vi "holonomic-drive-test.vi"() -> (3 "ALL TESTS PASSED":bool)   [LabVIEW 2019]
uses:
  <vilib>/Rock Robotics/WPI/ThirdParty/JAS_Junk/TrajLib/POSE2D.ctl
  <vilib>/Rock Robotics/WPI/ThirdParty/JAS_Junk/TrajLib/TRANSLATION2D.ctl
  <vilib>/Rock Robotics/WPI/ThirdParty/JAS_Junk/TrajLib/ROTATION2D.ctl
  <vilib>/Rock Robotics/WPI/ThirdParty/JAS_Junk/TrajLib/Translation_Create.vi
  <vilib>/Rock Robotics/WPI/ThirdParty/JAS_Junk/TrajLib/ProfiledPIDController_NewPeriod.vi
  <vilib>/Rock Robotics/WPI/ThirdParty/JAS_Junk/TrajLib/PIDController_NewPeriod.vi
  <vilib>/Rock Robotics/WPI/ThirdParty/JAS_Junk/TrajLib/ProfiledPIDController_Calculate_Meas_Goal.vi
  <vilib>/Rock Robotics/WPI/ThirdParty/JAS_Junk/TrajLib/ChassisSpeeds_FromFieldRelativeSpeeds.vi
  <vilib>/Rock Robotics/WPI/ThirdParty/JAS_Junk/TrajLib/PIDController_Reset.vi
  <vilib>/Rock Robotics/WPI/ThirdParty/JAS_Junk/TrajLib/PIDController_Calculate_SP_PV.vi
  <vilib>/Rock Robotics/WPI/ThirdParty/JAS_Junk/TrajLib/ProfiledPIDController_Reset_PosOnly.vi
  <vilib>/Rock Robotics/WPI/ThirdParty/JAS_Junk/TrajLib/Rotation_GetAngleCosSin.vi
  <vilib>/Rock Robotics/WPI/ThirdParty/JAS_Junk/TrajLib/Pose_RelativeTo.vi
  <vilib>/Rock Robotics/WPI/ThirdParty/JAS_Junk/TrajLib/Pose_getRotation.vi
  <vilib>/Rock Robotics/WPI/ThirdParty/JAS_Junk/TrajLib/Rotation_Minus.vi
  <vilib>/Rock Robotics/WPI/ThirdParty/JAS_Junk/TrajLib/TrapProfState_New.vi
  <vilib>/Rock Robotics/SystemInterfaces/NetworkCommunication/NetComm_UsageReport_report.vi
  <vilib>/Rock Robotics/WPI/ThirdParty/JAS_Junk/TrajLib/ProfiledPIDController_SetGoal_PosOnly.vi
  <vilib>/Rock Robotics/WPI/ThirdParty/JAS_Junk/TrajLib/ProfiledPIDController_Calculate_Meas.vi
  <vilib>/Rock Robotics/WPI/ThirdParty/JAS_Junk/TrajLib/Rotation_GetCos.vi
  <vilib>/Rock Robotics/WPI/ThirdParty/JAS_Junk/TrajLib/Rotation_GetSin.vi
  <vilib>/Rock Robotics/WPI/ThirdParty/JAS_Junk/TrajLib/ChassisSpeeds_New.vi
  <vilib>/Rock Robotics/WPI/ThirdParty/JAS_Junk/TrajLib/PIDController_SetSetpoint.vi
  <vilib>/Rock Robotics/WPI/ThirdParty/JAS_Junk/TrajLib/PIDController_Calculate_PV.vi
  <vilib>/Rock Robotics/WPI/ThirdParty/JAS_Junk/TrajLib/ProfiledPIDController_Reset.vi
  <vilib>/Rock Robotics/WPI/ThirdParty/JAS_Junk/TrajLib/Transform_Create_PosePose.vi
  <vilib>/Rock Robotics/WPI/ThirdParty/JAS_Junk/TrajLib/Pose_New_TRRO.vi
  <vilib>/Rock Robotics/WPI/ThirdParty/JAS_Junk/TrajLib/Rotation_UnaryMinus.vi
  <vilib>/Rock Robotics/WPI/ThirdParty/JAS_Junk/TrajLib/Rotation_RotateBy.vi
  <vilib>/Rock Robotics/WPI/ThirdParty/JAS_Junk/TrajLib/ProfiledPIDController_SetGoal.vi
  <vilib>/Rock Robotics/WPI/ThirdParty/JAS_Junk/TrajLib/TrapProfile_New.vi
  <vilib>/Rock Robotics/WPI/ThirdParty/JAS_Junk/TrajLib/ProfiledPIDController_GetPeriod.vi
  <vilib>/Rock Robotics/WPI/ThirdParty/JAS_Junk/TrajLib/TrapProfile_Calculate.vi
  <vilib>/Rock Robotics/WPI/ThirdParty/JAS_Junk/TrajLib/ControllerUtil_GetModulusError.vi
  <vilib>/Rock Robotics/WPI/ThirdParty/JAS_Junk/TrajLib/Translation_RotateBy.vi
  <vilib>/Rock Robotics/WPI/ThirdParty/JAS_Junk/TrajLib/Translation_Minus.vi
  <vilib>/Rock Robotics/WPI/ThirdParty/JAS_Junk/TrajLib/Rotation_CreateXY.vi
  <vilib>/Rock Robotics/WPI/ThirdParty/JAS_Junk/TrajLib/TrapProfile_ShouldFlipAcceleration.vi
  <vilib>/Rock Robotics/WPI/ThirdParty/JAS_Junk/TrajLib/TrapProfile_Direct.vi
  <vilib>/Rock Robotics/WPI/ThirdParty/JAS_Junk/TrajLib/PIDController_GetPeriod.vi
  <vilib>/Rock Robotics/WPI/ThirdParty/JAS_Junk/TrajLib/Util_CalcDist.vi
  <vilib>/Rock Robotics/WPI/ThirdParty/JAS_Junk/TrajLib/Util_LibraryGlobals.vi
  <vilib>/Rock Robotics/WPI/ThirdParty/JAS_Junk/TrajLib/Trajectory_Library.lvlib
panel:
  out "Test2 Passed":bool
  out "Test2 Omega":dbl
  out "Test2 Y":dbl
  out "Test2 X":dbl
  out "End Angle":dbl
  out "Y Err":dbl
  out "X err":dbl
  out "UpdatedPose":T1 {"ROTATION"."SIN" format="%13.4f"; "ROTATION"."COS" format="%13.4f"; "ROTATION"."VALUE" format="%13.4f"; "TRANSLATION"."Y" format="%14.3f"; "TRANSLATION"."X" format="%14.3f"}
  out "Init Pose":T1 {"ROTATION"."SIN" format="%13.4f"; "ROTATION"."COS" format="%13.4f"; "ROTATION"."VALUE" format="%13.4f"; "TRANSLATION"."Y" format="%14.3f"; "TRANSLATION"."X" format="%14.3f"}
  out "Traj Create Error":errorcluster
  out "Processing Timer Per Pass":dbl
  out "TotalTime":dbl
  out "TotalPasses":dbl
  out "Test Passed":bool
  out "TotalTImeSecs":dbl
  out "Position Graph":cluster{dbl[], dbl[]}[](graph)
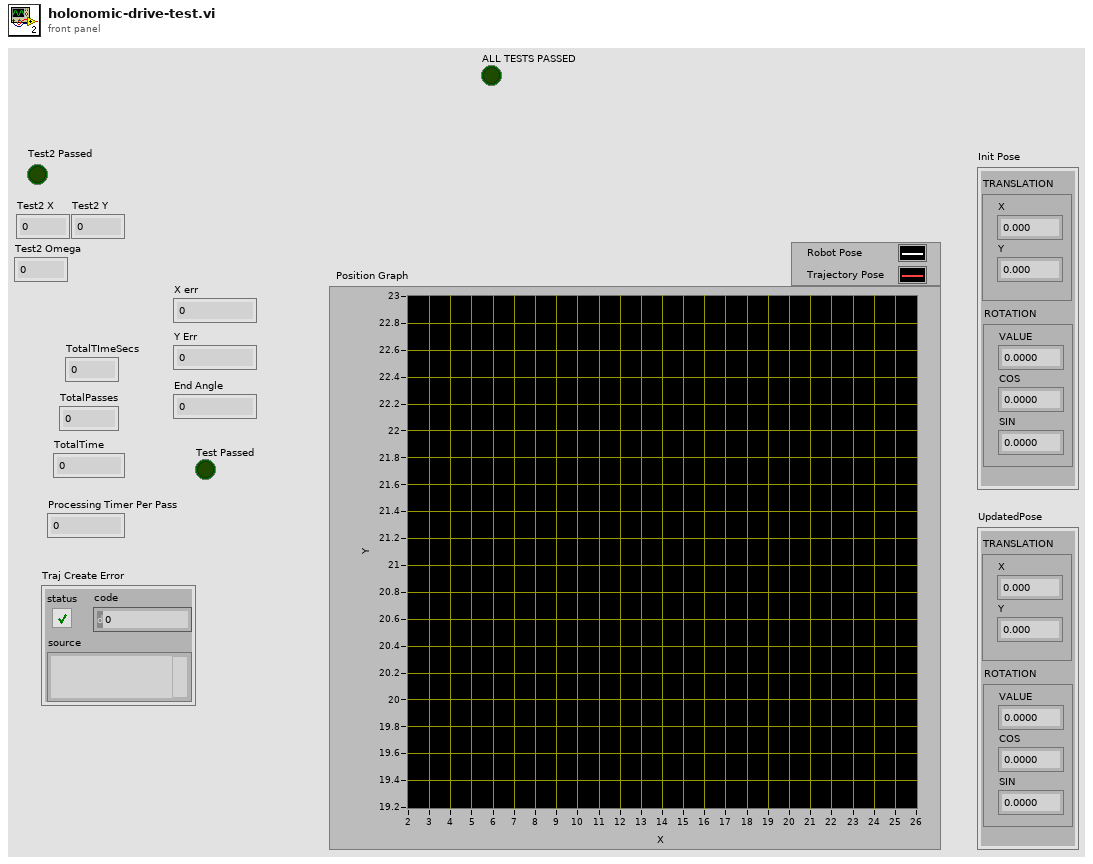
[diagram p1: front panel]
types:
  T1 = typedef "Trajectory_Library.lvlib/POSE2D.ctl" = cluster{"TRANSLATION":T2, "ROTATION":T3}
  T2 = typedef "Trajectory_Library.lvlib/TRANSLATION2D.ctl" = cluster{"X":dbl, "Y":dbl}
  T3 = typedef "Trajectory_Library.lvlib/ROTATION2D.ctl" = cluster{"VALUE":dbl, "COS":dbl, "SIN":dbl}
  T4 = typedef "Trajectory_Library.lvlib/TRAPEZOID_PROFILE_CONSTRAINT.ctl" = cluster{"MaxVelocity":dbl, "MaxAcceleration":dbl}
  T5 = typedef "Trajectory_Library.lvlib/PID_CONTROLLER.ctl" = cluster{"Kp":dbl, "Ki":dbl, "Kd":dbl, "Period":dbl, "Max_Integral":dbl, "Min_Integral":dbl, "Max_Input":dbl, "Min_Input":dbl, "Continuous":bool, "PositionError":dbl, "VelocityError":dbl, "PrevError":dbl, "TotalError":dbl, "PositionTolerance":dbl, "VelocityTolerance":dbl, "SetPoint":dbl, "Kf":dbl, "Prev_Deriv":dbl, "Prev_Deriv 2":dbl, "DerivativeFilter":bool, "Min_Output":dbl, "Max_Output":dbl, "Prev_F_P":dbl, "Prev_F_P_2":dbl, "AntiWindupActive":bool, "Measurement":dbl}
  T6 = typedef "Trajectory_Library.lvlib/PROFILED_PID_CONTROLLER.ctl" = cluster{"Controller":T5, "Goal":T7, "Setpoint":T7, "Constraint":T4}
  T7 = typedef "Trajectory_Library.lvlib/TRAPEZOID_PROFILE_STATE.ctl" = cluster{"Position":dbl, "Velocity":dbl}
  T8 = typedef "Trajectory_Library.lvlib/TRAJ_CONFIG.ctl" = cluster{"MaxVelocity":dbl, "Max Acceleration":dbl, "StartVelocity":dbl, "End Velocity":dbl, "Reversed":bool, "DiffDrKineConstntDefined":bool, "CentAcellConstntDefined":bool, "DiffDrVoltConstntDefined":bool, "DIFF_DRIVE_KINE_CONSTRAINT":T9, "CENTRIPETAL_ACCEL_CONSTRAINT":T11, "SwerveDrKineConstntDefined":bool, "SWERVE_DRIVE_KINE_CONSTRAINT":T12, "DIFF_DRIVE_VOLTAGE_CONSTRAINT":T15, "MECANUM_DRIVE_KINE_CONSTRAINT":T17, "MecanumDrKineConstntDefined":bool}
  T9 = typedef "Trajectory_Library.lvlib/TRAJ_CONSTRAINT_DIIF_DRIVE_KINEMATICS.ctl" = cluster{"Max Speed (M/S)":dbl, "DIFF_DRIVE_KINEMATICS":T10}
  T10 = typedef "Trajectory_Library.lvlib/DIFF_DRIVE_KINEMATICS.ctl" = cluster{"TrackWidth_Meters":dbl}
  T11 = typedef "Trajectory_Library.lvlib/TRAJ_CONSTRAINT_CENTRIPETAL_ACCEL.ctl" = cluster{"Max Cent Accel":dbl}
  T12 = typedef "Trajectory_Library.lvlib/TRAJ_CONSTRAINT_SWERVE_DRIVE_KINEMATICS.ctl" = cluster{"Max Speed (M/S)":dbl, "SwerveKinematics":T13}
  T13 = typedef "Trajectory_Library.lvlib/SWERVE_DRIVE_KINEMATICS.ctl" = cluster{"NumModules":i32, "InverseKinematics":T14, "ForwardKinematics":T14, "Modules":T2[], "PrevCoR":T2}
  T14 = typedef "NI_Matrix.lvlib/RealMatrix.ctl" = dbl[][]
  T15 = typedef "Trajectory_Library.lvlib/TRAJ_CONSTRAINT_DIIF_DRIVE_VOLTAGE.ctl" = cluster{"Max Voltage":dbl, "DIFF_DRIVE_KINEMATICS":T10, "SIMPLE_MOTOR_FF":T16}
  T16 = typedef "Trajectory_Library.lvlib/SIMPLE_MOTOR_FF.ctl" = cluster{"Ks":dbl, "Kv":dbl, "Ka":dbl}
  T17 = typedef "Trajectory_Library.lvlib/TRAJ_CONSTRAINT_MECA_DRIVE_KINEMATICS.ctl" = cluster{"Max Speed (M/S)":dbl, "MECA_DRIVE_KINEMATICS":T18}
  T18 = typedef "Trajectory_Library.lvlib/MECA_DRIVE_KINEMATICS.ctl" = cluster{"FrontLeft":T2, "FrontRight":T2, "RearLeft":T2, "RearRight":T2, "InverseKinematics":T14, "ForwardKinematics":T14, "PrevCoR":T2}
  T19 = typedef "Trajectory_Library.lvlib/HOLONOMIC_DRV_CTRL.ctl" = cluster{"poseTolerance":T1, "poseError":T1, "Enabled":bool, "PID_xCtrl":T5, "PID_yCtrl":T5, "PROF_PID_thetaCtrl":T6, "RotationError":T3, "FirstRun":bool}
  T20 = typedef "Trajectory_Library.lvlib/TRAJECTORY.ctl" = cluster{"TotalTImeSecs":dbl, "States":T21[]}
  T21 = typedef "Trajectory_Library.lvlib/TRAJ_STATE.ctl" = cluster{"TimeSeconds":dbl, "Velocity":dbl, "Acceleration":dbl, "POSE":T1, "Curvature":dbl}
  T22 = typedef "Trajectory_Library.lvlib/CHASSIS_SPEEDS.ctl" = cluster{"vX":dbl, "vY":dbl, "vOmega":dbl}
  T23 = typedef "Trajectory_Library.lvlib/TWIST2D.ctl" = cluster{"dX":dbl, "dY":dbl, "dTHETA":dbl}
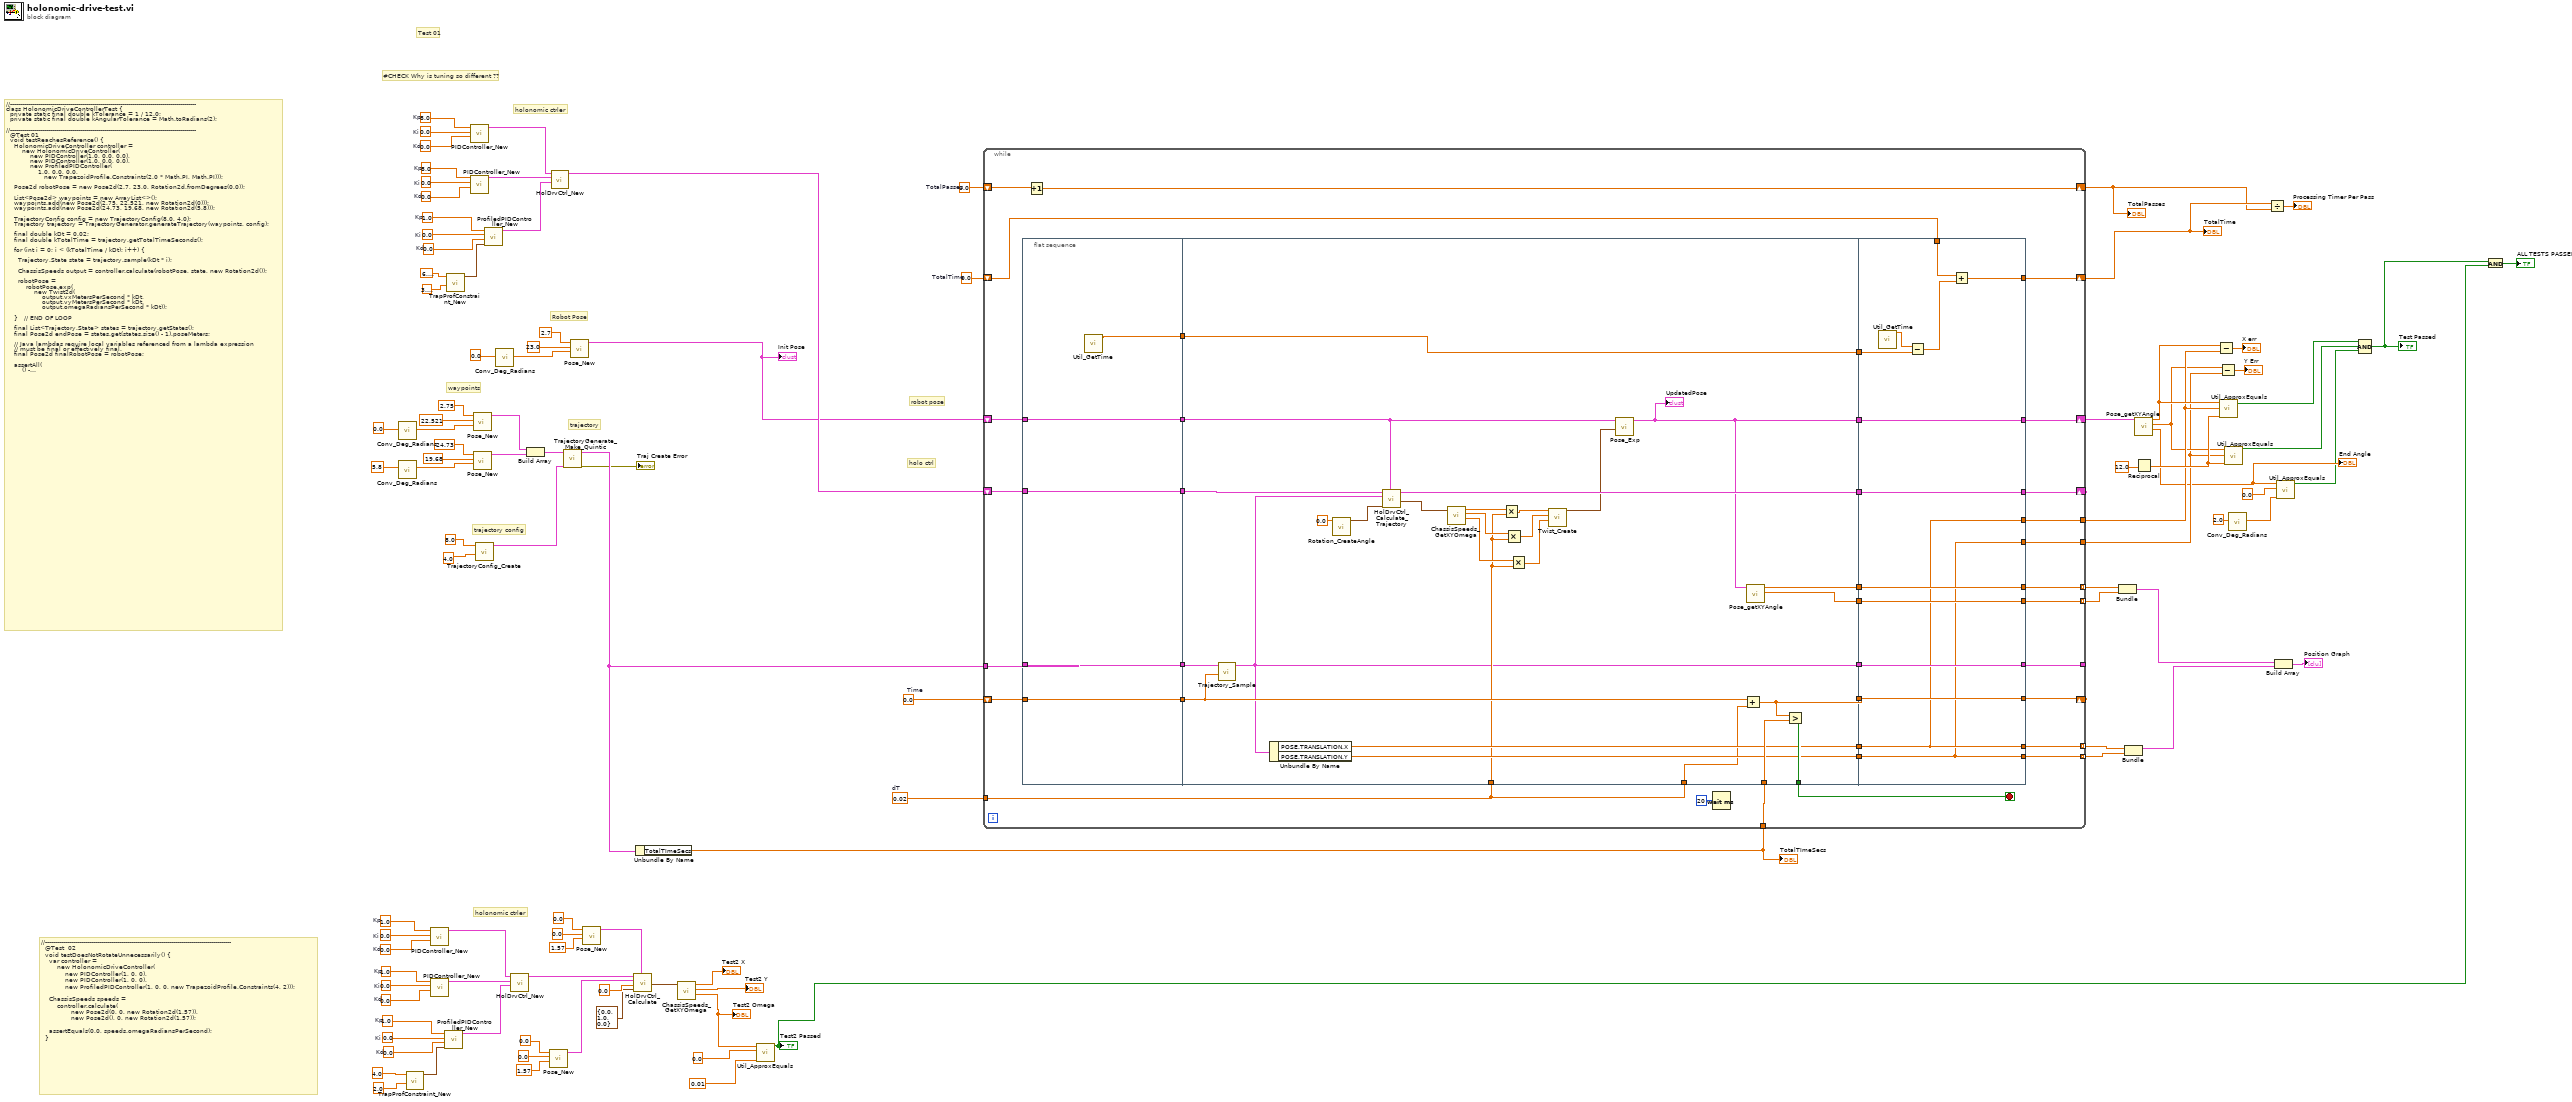
[diagram p0: block diagram]
diagram:
  w22 = 1.0  # Kp
  w23 = 0.0  # Ki
  w24 = 0.0  # Kd
  w28 = 1.0  # Kp
  w29 = 0.0  # Ki
  w30 = 0.0  # Kd
  w31 = 1.0  # Kp
  w32 = 0.0  # Ki
  w33 = 0.0  # Kd
  w55 = 0.02  # dT
  w64 = 1.0  # Kp
  w65 = 0.0  # Ki
  w66 = 0.0  # Kd
  w70 = 8.0  # Kp
  w71 = 0.0  # Ki
  w72 = 0.0  # Kd
  w73 = 8.0  # Kp
  w74 = 0.0  # Ki
  w75 = 0.0  # Kd
  w79 = 0.0  # TotalPasses
  w80 = 0.0  # TotalTime
  w89 = 0.0  # Time
  # "holonomic ctrler"
  # "//---------------------------------------------------------------------------------------------\n  @Test  02\n  void testDoesNotRotateUnnecessarily() {\n    var controller =\n        new HolonomicDriveController(\n            new PIDController(1, 0, 0),\n            new PIDController(1, 0, 0),\n            new ProfiledPIDController(1, 0, 0, new TrapezoidProfile.Constraints(4, 2)));\n\n    ChassisSpeeds speeds =\n        controller.calculate(\n               new Pose2d(0, 0, new Rotation2d(1.57)), \n               new Pose2d(), 0, new Rotation2d(1.57));\n\n    assertEquals(0.0, speeds.omegaRadiansPerSecond);\n  }"
  # "#CHECK Why is tuning so different ??"
  # "robot pose"
  # "holo ctrl"
  # "holonomic ctrler"
  # "Test 01"
  # "Robot Pose"
  # "//---------------------------------------------------------------------------------------------\nclass HolonomicDriveControllerTest {\n  private static final double kTolerance = 1 / 12.0;\n  private static final double kAngularTolerance = Math.toRadians(2);\n\n//---------------------------------------------------------------------------------------------\n  @Test 01\n  void testReachesReference() {\n    HolonomicDriveController controller =\n        new HolonomicDriveController(\n            new PIDController(1.0, 0.0, 0.0),\n            new PIDController(1.0, 0.0, 0.0),\n            new ProfiledPIDController(\n                1.0, 0.0, 0.0, \n                   new TrapezoidProfile.Constraints(2.0 * Math.PI, Math.PI)));\n\n    Pose2d robotPose = new Pose2d(2.7, 23.0, Rotation2d.fromDegrees(0.0));\n\n    List<Pose2d> waypoints = new ArrayList<>();\n    waypoints.add(new Pose2d(2.75, 22.521, new Rotation2d(0)));\n    waypoints.add(new Pose2d(24.73, 19.68, new Rotation2d(5.8)));\n\n    TrajectoryConfig config = new TrajectoryConfig(8.0, 4.0);\n    Trajectory trajectory = TrajectoryGenerator.generateTrajectory(waypoints, config);\n\n    final double kDt = 0.02;\n    final double kTotalTime = trajectory.getTotalTimeSeconds();\n\n    for (int i = 0; i < (kTotalTime / kDt); i++) {\n\n      Trajectory.State state = trajectory.sample(kDt * i);\n\n      ChassisSpeeds output = controller.calculate(robotPose, state, new Rotation2d());\n\n      robotPose =\n          robotPose.exp(\n              new Twist2d(\n                  output.vxMetersPerSecond * kDt,\n                  output.vyMetersPerSecond * kDt,\n                  output.omegaRadiansPerSecond * kDt));\n\n    }   // END OF LOOP\n\n    final List<Trajectory.State> states = trajectory.getStates();\n    final Pose2d endPose = states.get(states.size() - 1).poseMeters;\n\n    // Java lambdas require local variables referenced from a lambda expression\n    // must be final or effectively final.\n    final Pose2d finalRobotPose = robotPose;\n\n    assertAll(\n        () -> assertEquals(endPose.getX(), finalRobotPose.getX(), kTolerance),\n        () -> assertEquals(endPose.getY(), finalRobotPose.getY(), kTolerance),\n        () ->\n            assertEquals(\n                0.0,\n                MathUtil.angleModulus(finalRobotPose.getRotation().getRadians()),\n                kAngularTolerance));\n  }\n}"
  # "trajectory config"
  # "trajectory"
  # "waypoints"
  n1 = call <vilib>:"Conv_Deg_Radians.vi"("Degress"=0.0 ("Heading")) -> ("Radians"=w93:dbl)  [unwired: 10 in]
  n2 = call <vilib>:"Conv_Deg_Radians.vi"("Degress"=5.8 ("Heading")) -> ("Radians"=w97:dbl)  [unwired: 10 in]
  n3 = call <vilib>:"TrapProfConstraint_New.vi"("Max Accel"=2.0, "Max Speed (M/S)"=4.0) -> ("TRAPEZOID_PROFILE_CONSTRAINT"=w25:T4)  [unwired: 9 in]
  n4 = call <vilib>:"PIDController_New.vi"("Kd"=w33, "Ki"=w32, "Kp"=w31) -> ("PID_CONTROLLER"=w27:T5)  [unwired: 8 in]
  n5 = call <vilib>:"PIDController_New.vi"("Kd"=w30, "Ki"=w29, "Kp"=w28) -> ("PID_CONTROLLER"=w26:T5)  [unwired: 8 in]
  n6 = call <vilib>:"ProfiledPIDController_New.vi"("Constraints"=w25, "Kd"=w24, "Ki"=w23, "Kp"=w22) -> ("PROFILED_PID_CONTROLLER"=w21:T6)  [unwired: 7 in]
  n7 = call <vilib>:"TrapProfConstraint_New.vi"("Max Accel"=3.141592653589793, "Max Speed (M/S)"=6.283185307179586) -> ("TRAPEZOID_PROFILE_CONSTRAINT"=w67:T4)  [unwired: 9 in]
  n8 = call <vilib>:"PIDController_New.vi"("Kd"=w75, "Ki"=w74, "Kp"=w73) -> ("PID_CONTROLLER"=w69:T5)  [unwired: 8 in]
  n9 = call <vilib>:"PIDController_New.vi"("Kd"=w72, "Ki"=w71, "Kp"=w70) -> ("PID_CONTROLLER"=w68:T5)  [unwired: 8 in]
  n10 = call <vilib>:"Pose_New.vi"("Heading"=w93, "Y"=22.521, "X"=2.75) -> ("out POSe"=w92:T1)  [unwired: 8 in]
  n11 = call <vilib>:"Pose_New.vi"("Heading"=w97, "Y"=19.68, "X"=24.73) -> ("out POSe"=w90:T1)  [unwired: 8 in]
  n12 = call <vilib>:"TrajectoryConfig_Create.vi"("MaxAcceleration"=4.0, "MaxVelocity"=8.0) -> ("TRAJECTORY_CONFIG"=w101:T8)  [unwired: 9 in]
  n13 = call <vilib>:"ProfiledPIDController_New.vi"("Constraints"=w67, "Kd"=w66, "Ki"=w65, "Kp"=w64) -> ("PROFILED_PID_CONTROLLER"=w63:T6)  [unwired: 7 in]
  n14 = call <vilib>:"Conv_Deg_Radians.vi"("Degress"=0.0 ("Heading")) -> ("Radians"=w57:dbl)  [unwired: 10 in]
  n15 = call <vilib>:"HolDrvCtrl_New.vi"("thetaProfiledPID_CTRL"=w21, "yPID_CTRL"=w26, "xPID_CTRL"=w27) -> ("outHOLONOMIC_DRV_CTRL"=w18:T19)  [unwired: 8 in]
  n16 = Build Array(w92, w90) -> (w102:T1[])
  n17 = call <vilib>:"Pose_New.vi"("Heading"=1.57, "Y"=0.0, "X"=0.0) -> ("out POSe"=w11:T1)  [unwired: 8 in]
  n18 = call <vilib>:"HolDrvCtrl_New.vi"("thetaProfiledPID_CTRL"=w63, "yPID_CTRL"=w68, "xPID_CTRL"=w69) -> ("outHOLONOMIC_DRV_CTRL"=w54:T19)  [unwired: 8 in]
  n19 = call <vilib>:"TrajectoryGenerate_Make_Quintic.vi"("traj_config"=w101, "waypointPOSE"=w102) -> ("error out"=→"Traj Create Error":errorcluster, "TRAJECTORY"=w88:T20)  [unwired: 8 in]
  n20 = call <vilib>:"Pose_New.vi"("Heading"=w57, "Y"=23.0, "X"=2.7) -> ("out POSe"=w53:T1)  [unwired: 8 in]
  "Init Pose" <- w53
  n21 = call <vilib>:"Pose_New.vi"("Heading"=1.57, "Y"=0.0, "X"=0.0) -> ("out POSe"=w10:T1)  [unwired: 8 in]
  n22 = call <vilib>:"HolDrvCtrl_Calculate.vi"("currentPose"=w10, "angleRef"=T3 {"VALUE"=0.0, "COS"=1.0, "SIN"=0.0}, "linearVelRef"=0.0, "poseRef"=w11, "inHOLONOMIC_DRV_CTRL"=w18) -> ("calcChassisSpeed"=w7:T22)  [unwired: 5 in, 1 out]
  n23 = Unbundle By Name(w88) -> ("TotalTImeSecs"=w81:dbl)
  "TotalTImeSecs" <- w81
  n24 = call <vilib>:"ChassisSpeeds_GetXYOmega.vi"("CHASSIS"=w7) -> ("vAngular"=w4:dbl, "vY"=→"Test2 Y":dbl, "vX"=→"Test2 X":dbl)  [unwired: 8 in]
  "Test2 Omega" <- w4
  n25 = call <vilib>:"Util_ApproxEquals.vi"("Tolerance"=0.01, "Value 2"=0.0, "Value 1"=w4) -> ("ApproxEquals"=w2:bool)  [unwired: 8 in]
  "Test2 Passed" <- w2
  n26 = while {
    shift-right: [w139] -> _
    shift-left: w89 -> [w136]
    tunnel: w88 -> [w137]
    tunnel: w81 -> [w138]
    tunnel: [w135] -> w87 mode=indexing
    tunnel: [w134] -> w86 mode=indexing
    tunnel: [w133] -> w84 mode=indexing
    tunnel: [w132] -> w83 mode=indexing
    shift-right: [w121] -> w78
    shift-left: w80 -> [w120]
    shift-right: [w118] -> w77
    shift-left: w79 -> [w119]
    tunnel: w55 -> [w110]
    shift-right: [w112] -> _
    shift-left: w54 -> [w116]
    shift-right: [w109] -> w51
    shift-left: w53 -> [w113]
    tunnel: [w107] -> _
    tunnel: [w105] -> w47
    tunnel: [w104] -> w45
    stop <- w131 stop-if-true
    n27 = flat-sequence {
      tunnel: w136 -> [w143]
      tunnel: w137 -> [w144]
      tunnel: [w144] -> w130
      tunnel: [w143] -> w129
      tunnel: [w142] -> w123
      tunnel: w116 -> [w141]
      tunnel: [w141] -> w115
      tunnel: [w140] -> w114
      tunnel: w113 -> [w140]
      tunnel: [w171] -> w131
      tunnel: w138 -> [w169]
      tunnel: w130 -> [w168]
      tunnel: w129 -> [w167]
      tunnel: [w170] -> w128
      tunnel: [w150] -> w127
      tunnel: [w149] -> w126
      tunnel: [w166] -> w125
      tunnel: [w165] -> w124
      tunnel: w123 -> [w164]
      tunnel: [w164] -> w122
      tunnel: w110 -> [w163]
      tunnel: w115 -> [w162]
      tunnel: w114 -> [w160]
      tunnel: [w161] -> w111
      tunnel: w110 -> [w155]
      tunnel: [w148] -> w108
      tunnel: [w147] -> w106
      tunnel: [w173] -> w132
      tunnel: [w172] -> w133
      tunnel: [w182] -> w134
      tunnel: [w183] -> w135
      tunnel: [w184] -> w139
      tunnel: w128 -> [w184]
      tunnel: w127 -> [w183]
      tunnel: w126 -> [w182]
      tunnel: w125 -> [w172]
      tunnel: w124 -> [w173]
      tunnel: w122 -> [w180]
      tunnel: [w179] -> w121
      tunnel: w120 -> [w177]
      tunnel: [w176] -> w112
      tunnel: w111 -> [w176]
      tunnel: [w175] -> w109
      tunnel: w108 -> [w175]
      tunnel: [w174] -> w107
      tunnel: w106 -> [w174]
      tunnel: [w173] -> w105
      tunnel: [w172] -> w104
      frame #0 {
        n28 = call <vilib>:"Util_GetTime.vi"() -> ("FPGA_Time_Seconds"=w142:dbl)  [unwired: 10 in, 1 out]
      }
      frame #1 {
        n29 = call <vilib>:"Trajectory_Sample.vi"("Time"=w167, "InputTRAJECTORY"=w168) -> ("OutputTRAJ_STATE"=w147:T21)  [unwired: 9 in]
        n30 = Unbundle By Name(w147) -> ("POSE.TRANSLATION.X"=w165:dbl, "POSE.TRANSLATION.Y"=w166:dbl)
        n31 = call <vilib>:"Rotation_CreateAngle.vi"("Angle"=0.0) -> ("ROTATION"=w145:T3)  [unwired: 10 in]
        n32 = call <vilib>:"HolDrvCtrl_Calculate_Trajectory.vi"("currentPose"=w160, "angleRef"=w145, "desiredTrajState"=w147, "inHOLONOMIC_DRV_CTRL"=w162) -> ("calcChassisSpeed"=w159:T22, "outHOLONOMIC_DRV_CTRL"=w161:T19)  [unwired: 6 in]
        n33 = call <vilib>:"ChassisSpeeds_GetXYOmega.vi"("CHASSIS"=w159) -> ("vAngular"=w156:dbl, "vY"=w157:dbl, "vX"=w158:dbl)  [unwired: 8 in]
        n34 = Multiply(x=w158, y=w155) -> (x*y=w154:dbl)
        n35 = Multiply(x=w157, y=w155) -> (x*y=w153:dbl)
        n36 = Multiply(x=w156, y=w155) -> (x*y=w152:dbl)
        n37 = call <vilib>:"Twist_Create.vi"("dTHETA"=w152, "dY"=w153, "dX"=w154) -> ("TWIST"=w151:T23)  [unwired: 8 in]
        n38 = call <vilib>:"Pose_Exp.vi"("TWIST"=w151, "POSE"=w160) -> ("UpdatedPose"=w148:T1)  [unwired: 9 in]
        "UpdatedPose" <- w148
        n39 = Add(x=w167, y=w163) -> (x+y=w170:dbl)
        n40 = call <vilib>:"Pose_getXYAngle.vi"("in POSE"=w148) -> ("Y"=w149:dbl, "X"=w150:dbl)  [unwired: 8 in, 1 out]
        n41 = Greater?(x=w170, y=w169) -> (0:w171:bool)
      }
      frame #2 {
        n42 = call <vilib>:"Util_GetTime.vi"() -> ("FPGA_Time_Seconds"=w181:dbl)  [unwired: 10 in, 1 out]
        n43 = Subtract(x=w181, y=w180) -> (x-y=w178:dbl)
        n44 = Add(x=w177, y=w178) -> (x+y=w179:dbl)
      }
    }
    n45 = Increment(x=w119) -> (x+1=w118:dbl)
    n46 = Wait (ms)(milliseconds to wait=u32 20) -> ()  [unwired: 1 out]
  }
  "TotalPasses" <- w77
  "TotalTime" <- w78
  n47 = Bundle(w87, w86) -> (w52:cluster{dbl[], dbl[]})  [unwired: 1 in]
  n48 = Bundle(w83, w84) -> (w82:cluster{dbl[], dbl[]})  [unwired: 1 in]
  n49 = call <vilib>:"Pose_getXYAngle.vi"("in POSE"=w51) -> ("Angle"=w40:dbl, "Y"=w46:dbl, "X"=w48:dbl)  [unwired: 8 in]
  "End Angle" <- w40
  n50 = Reciprocal(x=12.0) -> (1/x=w49:dbl)
  n51 = Subtract(x=w48, y=w47) -> (x-y=→"X err":dbl)
  n52 = Subtract(x=w46, y=w45) -> (x-y=→"Y Err":dbl)
  n53 = call <vilib>:"Util_ApproxEquals.vi"("Tolerance"=w49, "Value 2"=w47, "Value 1"=w48) -> ("ApproxEquals"=w42:bool)  [unwired: 8 in]
  n54 = call <vilib>:"Util_ApproxEquals.vi"("Tolerance"=w49, "Value 2"=w45, "Value 1"=w46) -> ("ApproxEquals"=w41:bool)  [unwired: 8 in]
  n55 = call <vilib>:"Conv_Deg_Radians.vi"("Degress"=2.0) -> ("Radians"=w37:dbl)  [unwired: 10 in]
  n56 = Divide(x=w78, y=w77) -> (x/y=→"Processing Timer Per Pass":dbl)
  n57 = Build Array(w52, w82) -> (→"Position Graph":cluster{dbl[], dbl[]}[])
  n58 = call <vilib>:"Util_ApproxEquals.vi"("Tolerance"=w37, "Value 2"=0.0, "Value 1"=w40) -> ("ApproxEquals"=w36:bool)  [unwired: 8 in]
  n59 = Compound Arithmetic op=AND(w42, w41, w36) -> (w34:bool)
  "Test Passed" <- w34
  n60 = And(x=w34, y=w2) -> (x .and. y?=→"ALL TESTS PASSED":bool)
